vi "LV9_1.vi"() -> ()   [LabVIEW 2016]
uses:
  <vilib>/imath/engines/lvmath2/RunTimeEngine/RangeToken/NIMS_Range.vi
  <instcachedir>/0/NIMS_Range_A7C094595B484CA7AF10685B02D808ED.lvgen/NIMS_Range_A7C094595B484CA7AF10685B02D808ED_001.vi
  <vilib>/imathl/engines/lvmath/Functions/Error Handling/Create Error.vi
  <vilib>/imath/engines/lvmath2/RunTimeEngine/ArithmeticOperatorToken/NIMS_ArithmeticOperator_rightdiv.vi
  <instcachedir>/0/NIMS_ArithmeticOperator_rightdiv_0403F5D95ED04A4080FE3DA43A6A83B7.lvgen/NIMS_ArithmeticOperator_rightdiv_0403F5D95ED04A4080FE3DA43A6A83B7_005.vi
  <vilib>/imath/engines/lvmath2/RunTimeEngine/IndexReplace/NIMS V(S)=S.vi
  <instcachedir>/0/NIMS V(S)=S_57E16554CB8B4B90AAB163894F717546.lvgen/NIMS V(S)=S_57E16554CB8B4B90AAB163894F717546_000.vi
  <vilib>/imath/engines/lvmath2/RunTimeEngine/ArithmeticOperatorToken/NIMS_ArithmeticOperator_times.vi
  <instcachedir>/0/NIMS_ArithmeticOperator_times_953B34F74CAC448FB707D816A29CC5F0.lvgen/NIMS_ArithmeticOperator_times_953B34F74CAC448FB707D816A29CC5F0_000.vi
  <instcachedir>/0/NIMS_Range_A7C094595B484CA7AF10685B02D808ED.lvgen/NIMS_Range_A7C094595B484CA7AF10685B02D808ED_000.vi
  <vilib>/imath/engines/lvmath2/RunTimeEngine/BuiltInFunctions/fft/NIMS_fft(GV).vi
  <instcachedir>/0/NIMS_fft(GV)_4C6467FC22F84E4BA42517A07EF978B0.lvgen/NIMS_fft(GV)_4C6467FC22F84E4BA42517A07EF978B0_000.vi
  <vilib>/imath/engines/lvmath2/RunTimeEngine/ErrorHandling/NIMS_Error From Error Code.vi
  <vilib>/imath/engines/lvmath2/RunTimeSupport/NIMS_Error if Not Equal.vi
  <instcachedir>/0/NIMS_Error if Not Equal_43252A79AD05436189442EC0C5E5AB8A.lvgen/NIMS_Error if Not Equal_43252A79AD05436189442EC0C5E5AB8A_001.vi
  <vilib>/imath/engines/lvmath2/RunTimeEngine/IndexRead/NIMS V(V).vi
  <instcachedir>/0/NIMS V(V)_298D9CB7BFEB42B8BC8D9C3C28AE8C70.lvgen/NIMS V(V)_298D9CB7BFEB42B8BC8D9C3C28AE8C70_000.vi
  <vilib>/imath/engines/lvmath2/RunTimeEngine/BuiltInFunctions/abs/NIMS_abs(signed).vi
  <instcachedir>/0/NIMS_abs(signed)_C4FCB8E6058B49B797C7C8D53CA5F6EC.lvgen/NIMS_abs(signed)_C4FCB8E6058B49B797C7C8D53CA5F6EC_006.vi
  <vilib>/imath/engines/lvmath2/RunTimeEngine/ErrorHandling/NIMS_Create Error From Enums.vi
  <vilib>/imath/engines/lvmath2/RunTimeEngine/NodeEndStatement/NIMS_NodeEndStatement_Output.vi
  <instcachedir>/0/NIMS_NodeEndStatement_Output_53EC0D466D134D7ABD903AC30B43404B.lvgen/NIMS_NodeEndStatement_Output_53EC0D466D134D7ABD903AC30B43404B_005.vi
  <instcachedir>/0/NIMS_NodeEndStatement_Output_53EC0D466D134D7ABD903AC30B43404B.lvgen/NIMS_NodeEndStatement_Output_53EC0D466D134D7ABD903AC30B43404B_004.vi
  <vilib>/imath/engines/lvmath2/RunTimeEngine/ErrorHandling/NIMS_Finalize Error.vi
panel:
  in  "Stop Button":bool
  in  "L":i32(slide) scale=10.0..20.0
  in  "Cutoff frequency":dbl(slide) scale=100.0..400.0
  out "Filter impulse response":cluster{"LL":i32[], "H":dbl[]}(graph)
  out "Filter frequency response":cluster{"f":dbl[], "FH":dbl[]}(graph)
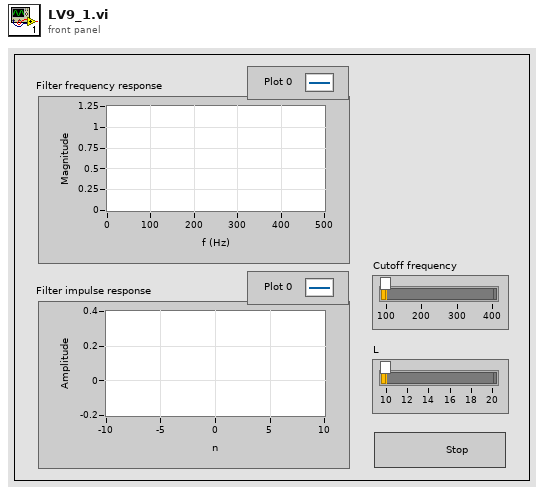
[diagram p1: front panel]
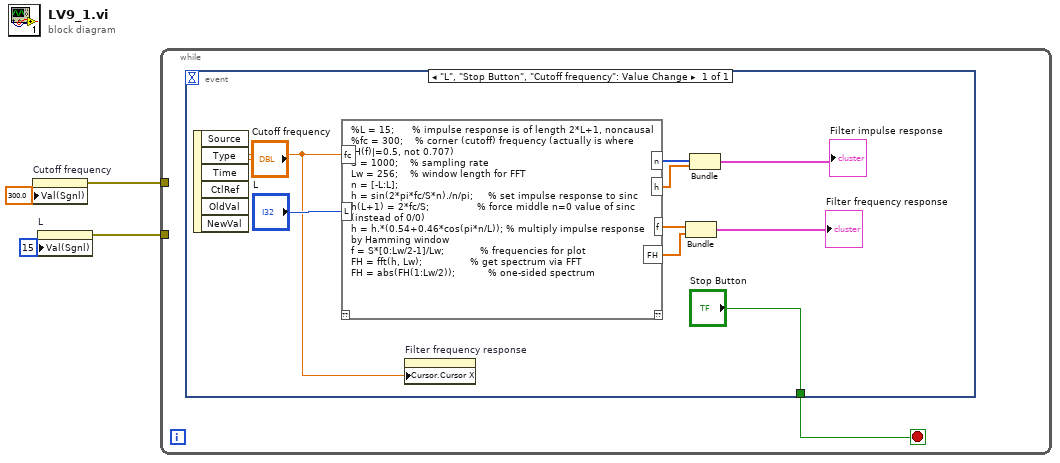
[diagram p0: block diagram]
diagram:
  n1 = property on="Cutoff frequency" class="Slide (strict)"("Val(Sgnl)"=300.0 ("Cutoff frequency")) -> (error out=w4:errorcluster)  [unwired: 2 in, 1 out]
  n2 = property on="L" class="Slide (strict)"("Val(Sgnl)"=15 ("L")) -> (error out=w2:errorcluster)  [unwired: 2 in, 1 out]
  n3 = while {
    tunnel: w4 -> [_]
    tunnel: w2 -> [_]
    stop <- w5 stop-if-true
    n4 = event shown="[0] \"L\", \"Stop Button\", \"Cutoff frequency\": Value Change" {
      selector: _ -> [_]
      dyn-events: _ -> [_]
      timeout: _ -> [_]
      tunnel: ["Stop Button"] -> w5
      event "L", "Stop Button", "Cutoff frequency": Value Change {
        n5 = event-data() -> ()  [unwired: 1 in, 6 out]
        n6 = mathscript code="%L = 15;      % impulse response is of length 2*L+1, noncausal\n%fc = 300;    % corner (cutoff) frequency (actually is where |H(f)|=0.5, not 0.707)\nS = 1000;    % sampling rate\nLw = 256;    % window length for FFT\nn = [-L:L];\nh = sin(2*pi*fc/S*n)./n/pi;     % set impulse response to sinc\nh(L+1) = 2*fc/S;                % force middle n=0 value of sinc (instead of 0/0)\nh = h.*(0.54+0.46*cos(pi*n/L)); % multiply impulse response by Hamming window\nf = S*[0:Lw/2-1]/Lw;            % frequencies for plot\nFH = fft(h, Lw);                % get spectrum via FFT\nFH = abs(FH(1:Lw/2));           % one-sided spectrum"("fc"="Cutoff frequency", "L"="L") -> ("FH"=w11:dbl[], "f"=w12:dbl[], "n"=w14:i32[], "h"=w13:dbl[])  [unwired: 1 in, 1 out]
        n7 = property on="Filter frequency response" class="XYGraph (strict)"("Cursor.Cursor X"="Cutoff frequency") -> ()  [unwired: 2 in, 2 out]
        n8 = Bundle("f"=w12, "FH"=w11) -> (→"Filter frequency response":cluster{"f":dbl[], "FH":dbl[]})  [unwired: 1 in]
        n9 = Bundle("n"=w14, "h"=w13) -> (→"Filter impulse response":cluster{"n":i32[], "h":dbl[]})  [unwired: 1 in]
      }
    }
  }
